vi "compliancesubvi2.vi"(2 "Value1":dbl, 3 "compliance (V)":dbl=0.0001 format="%^.2e", 4 "Mode":u16(ring)=4 items=["V", "I", "VPulse", "IPulse", "Common"], 5 "compliance (A)":dbl=0.0001 format="%^.2e") -> (0 "compliance":dbl, 1 "constant":dbl)   [LabVIEW 2012]
uses:
  Instance           1 24Saved   compliancesubvi2 .vi
  Instance           2 24Saved   compliancesubvi2 .vi
  Instance           3 24Saved   compliancesubvi2 .vi
  Instance           4 24Saved   compliancesubvi2 .vi
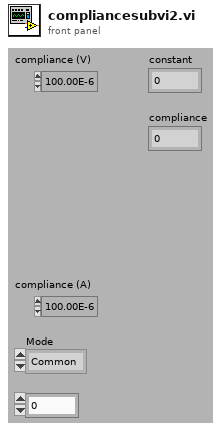
[diagram p1: front panel]
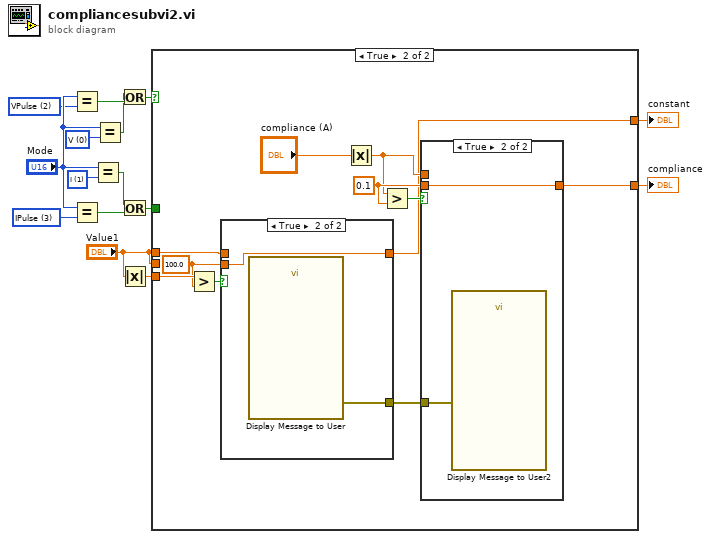
[diagram p0: block diagram]
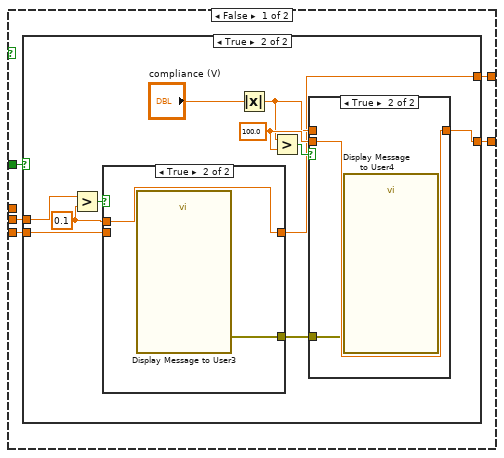
[diagram p2: hidden frame]
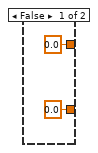
[diagram p3: hidden frame]
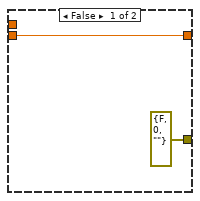
[diagram p4: hidden frame]
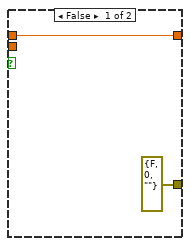
[diagram p6: hidden frame]
diagram:
  w13 = u16 3 items=["V", "I", "VPulse", "IPulse", "Common"] ("Mode")
  w12 = u16 1 items=["V", "I", "VPulse", "IPulse", "Common"] ("Mode")
  w7 = u16 2 items=["V", "I", "VPulse", "IPulse", "Common"] ("Mode")
  w5 = u16 0 items=["V", "I", "VPulse", "IPulse", "Common"] ("Mode")
  n1 = Equal?(x="Mode", y=w7) -> (x = y?=w8:bool)
  n2 = Equal?(x="Mode", y=w13) -> (x = y?=w11:bool)
  n3 = Equal?(x="Mode", y=w12) -> (x = y?=w10:bool)
  n4 = Equal?(x="Mode", y=w5) -> (x = y?=w6:bool)
  n5 = Or(x=w6, y=w8) -> (x .or. y?=w9:bool)
  n6 = Or(x=w10, y=w11) -> (x .or. y?=w4:bool)
  n7 = Absolute Value(x="Value1") -> (abs(x)=w15:dbl)
  n8 = case shown="True" w9 {
    tunnel: w15 -> [w19 w47]
    tunnel: "Value1" -> [_ w44]
    tunnel: w4 -> [w20 _]
    tunnel: "Value1" -> [w18 _]
    tunnel: [w17 w42] -> w2
    tunnel: [w16 w41] -> w1
    frame False {
      n9 = case shown="True" w20 {
        tunnel: w18 -> [_ w29]
        tunnel: w19 -> [_ w25]
        tunnel: [0.0 ("y") w24] -> w17
        tunnel: [0.0 ("y") w23] -> w16
        frame False {
        }
        frame True {
          w26 = 0.1 ("y")
          w32 = 100.0 ("y")
          n10 = Greater?(x=w29, y=w26) -> (0:w28:bool)
          n11 = case shown="True" w28 {
            tunnel: [errorcluster {"status"=FALSE, "code"=0, "source"=""} ("error out") w37] -> w27
            tunnel: [w34 w36] -> w24
            tunnel: w25 -> [w34 _]
            tunnel: w26 -> [_ w36]
            frame False {
            }
            frame True {
              n12 = call "Display Message to User3"() -> ("error out"=w37:errorcluster)  [unwired: 10 in, 1 out]
            }
          }
          n13 = Absolute Value(x="compliance (V)") -> (abs(x)=w30:dbl)
          n14 = Greater?(x=w30, y=w32) -> (0:w33:bool)
          n15 = case shown="True" w33 {
            tunnel: w30 -> [w38 _]
            tunnel: w32 -> [_ w40]
            tunnel: [w38 w40] -> w23
            tunnel: w27 -> [_ w39]
            frame False {
            }
            frame True {
              n16 = call "Display Message to User4"("error in (no error)"=w39) -> ()  [unwired: 9 in, 2 out]
            }
          }
        }
      }
    }
    frame True {
      w45 = 100.0 ("y")
      w50 = 0.1 ("y")
      n17 = Greater?(x=w47, y=w45) -> (0:w46:bool)
      n18 = case shown="True" w46 {
        tunnel: w45 -> [_ w55]
        tunnel: [w53 w55] -> w42
        tunnel: w44 -> [w53 _]
        tunnel: [errorcluster {"status"=FALSE, "code"=0, "source"=""} ("error out") w54] -> w43
        frame False {
        }
        frame True {
          n19 = call "Display Message to User"() -> ("error out"=w54:errorcluster)  [unwired: 10 in, 1 out]
        }
      }
      n20 = Absolute Value(x="compliance (A)") -> (abs(x)=w48:dbl)
      n21 = Greater?(x=w48, y=w50) -> (0:w51:bool)
      n22 = case shown="True" w51 {
        tunnel: w50 -> [_ w58]
        tunnel: [w56 w58] -> w41
        tunnel: w48 -> [w56 _]
        tunnel: w43 -> [_ w57]
        frame False {
        }
        frame True {
          n23 = call "Display Message to User2"("error in (no error)"=w57) -> ()  [unwired: 9 in, 2 out]
        }
      }
    }
  }
  "compliance" <- w1
  "constant" <- w2
